vi "solar_voy_def Import (Simple).vi"(4 "Default ID":u16, 5 "Endian (BIG)":enum8{"BIG", "LITTLE"}(ring), 6 "Suppress Errors? (T)":bool=TRUE, 7 "CMD":enum8{"CMD", "TLM"}(ring), 8 "error in (no error)":errorcluster, 9 "ITEMS (Simple)":T6[](array[typedef]), 10 "PACKET":string, 11 "TARGET":string) -> (0 "error out":errorcluster, 3 "PACKET":T1 {"last_time" format="%<%H:%M:%S%3u %m/%d/%y>T"})   [LabVIEW 2018]
uses:
  solar_voy_def_ctl MODIFIERS CONVERSION.ctl
  solar_voy_def_ctl MODIFIERS STATE.ctl
  solar_voy_def_ctl MODIFIERS UNITS.ctl
  solar_voy_def_ctl MODIFIERS LIMITS.ctl
  solar_voy_def_ctl MODIFIERS.ctl
  type/solar_type Item Type.ctl
  solar_voy_def_ctl ITEM TYPE.ctl
  solar_voy_def_ctl ITEM.ctl
  solar_voy_def_ctl PACKET_ID.ctl
  solar_voy_def_ctl PACKET.ctl
  solar_voy_def_ctl ITEM (Simple).ctl
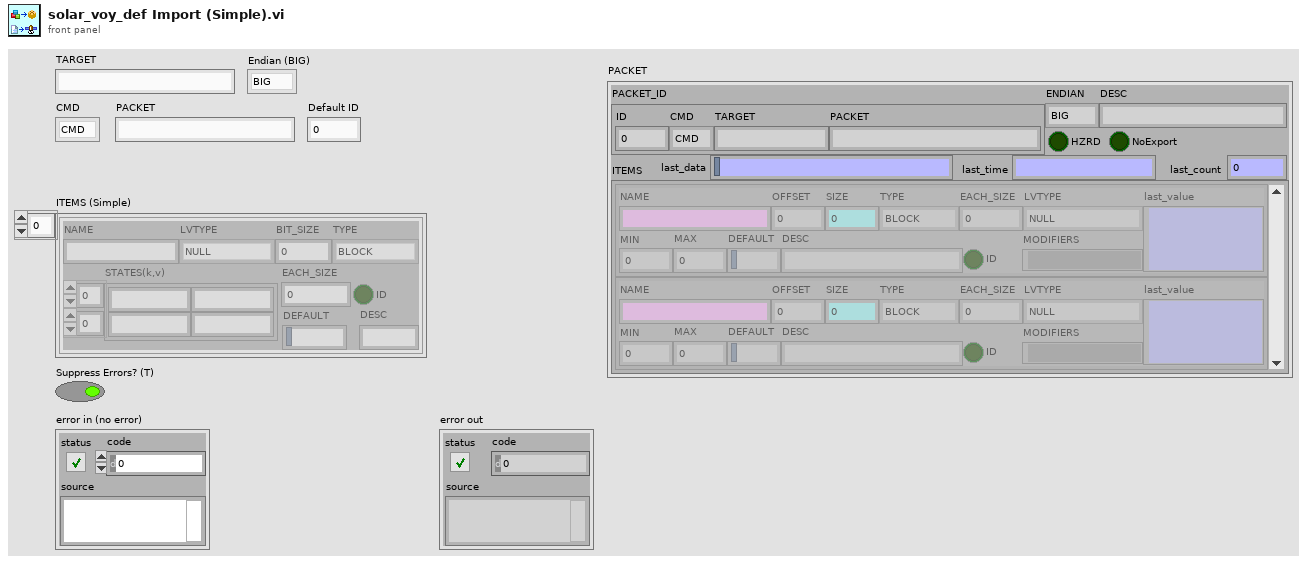
[diagram p1: front panel]
types:
  T1 = typedef "solar_voy_def_ctl PACKET.ctl" = cluster{"PACKET_ID":T2, "ENDIAN":enum8{"BIG", "LITTLE"}, "DESC":string, "HZRD":bool, "ITEMS":T3[], "NoExport":bool, "last_time":timestamp, "last_count":u32, "last_data":string}
  T2 = typedef "solar_voy_def_ctl PACKET_ID.ctl" = cluster{"ID":u16, "CMD":enum8{"CMD", "TLM"}, "TARGET":string, "PACKET":string}
  T3 = typedef "solar_voy_def_ctl ITEM.ctl" = cluster{"NAME":string, "OFFSET":i32, "SIZE":i32, "TYPE":T4, "EACH_SIZE":i32, "LVTYPE":T5, "MIN":dbl, "MAX":dbl, "DEFAULT":string, "DESC":string, "ID":bool, "MODIFIERS":variant, "last_value":variant}
  T4 = typedef "solar_voy_def_ctl ITEM TYPE.ctl" = enum8{"BLOCK", "INT", "UINT", "FLOAT", "STRING"}
  T5 = typedef "solar_type Item Type.ctl" = enum16{"NULL", "UNKNOWN", "CLUSTER", "I8", "I16", "I32", "I64", "U8", "U16", "U32", "U64", "U8_ENUM", "U16_ENUM", "U32_ENUM", "SGL", "DBL", "BOOLEAN", "STRING", "PATH", "VISA", "TAG", "TIME", "I8_1D", "I16_1D", "I32_1D", "I64_1D", "U8_1D", "U16_1D", "U32_1D", "U64_1D", "U8_ENUM_1D", "U16_ENUM_1D", "U32_ENUM_1D", "SGL_1D", "DBL_1D", "BOOLEAN_1D", "STRING_1D", "PATH_1D", "VISA_1D", "TAG_1D", "TIME_1D", "I8_2D", "I16_2D", "I32_2D", "I64_2D", "U8_2D", "U16_2D", "U32_2D", "U64_2D", "U8_ENUM_2D", "U16_ENUM_2D", "U32_ENUM_2D", "SGL_2D", "DBL_2D", "BOOLEAN_2D", "STRING_2D", "PATH_2D", "VISA_2D", "TAG_2D", "TIME_2D"}
  T6 = typedef "solar_voy_def_ctl ITEM (Simple).ctl" = cluster{"NAME":string, "LVTYPE":T5, "BIT_SIZE":i32, "TYPE":T4, "DEFAULT":string, "EACH_SIZE":i32, "ID":bool, "STATES(k,v)":string[][], "DESC":string}
  T7 = typedef "solar_voy_def_ctl MODIFIERS.ctl" = cluster{"LIMITS":T8, "UNITS":T9, "STATES":T10[], "CONVERSION":T11, "FORMAT":string, "REQUIRED":bool, "META":string[][]}
  T8 = typedef "solar_voy_def_ctl MODIFIERS LIMITS.ctl" = cluster{"NAME":string, "PERSIST":i32, "EN":bool, "RED_LO":dbl, "YEL_LO":dbl, "YEL_HI":dbl, "RED_HI":dbl, "GRN_LO":dbl, "GRN_HI":dbl, "FILENAME":string, "ARGS":string}
  T9 = typedef "solar_voy_def_ctl MODIFIERS UNITS.ctl" = cluster{"FULL":string, "ABV":string}
  T10 = typedef "solar_voy_def_ctl MODIFIERS STATE.ctl" = cluster{"KEY":string, "VALUE":string, "COLOR":string, "DESC":string, "HZRD":bool}
  T11 = typedef "solar_voy_def_ctl MODIFIERS CONVERSION.ctl" = cluster{"GENERIC":string, "FILENAME":string, "ARGS":string, "POLYS":cluster{"SEG":bool, "POLY":dbl[]}[]}
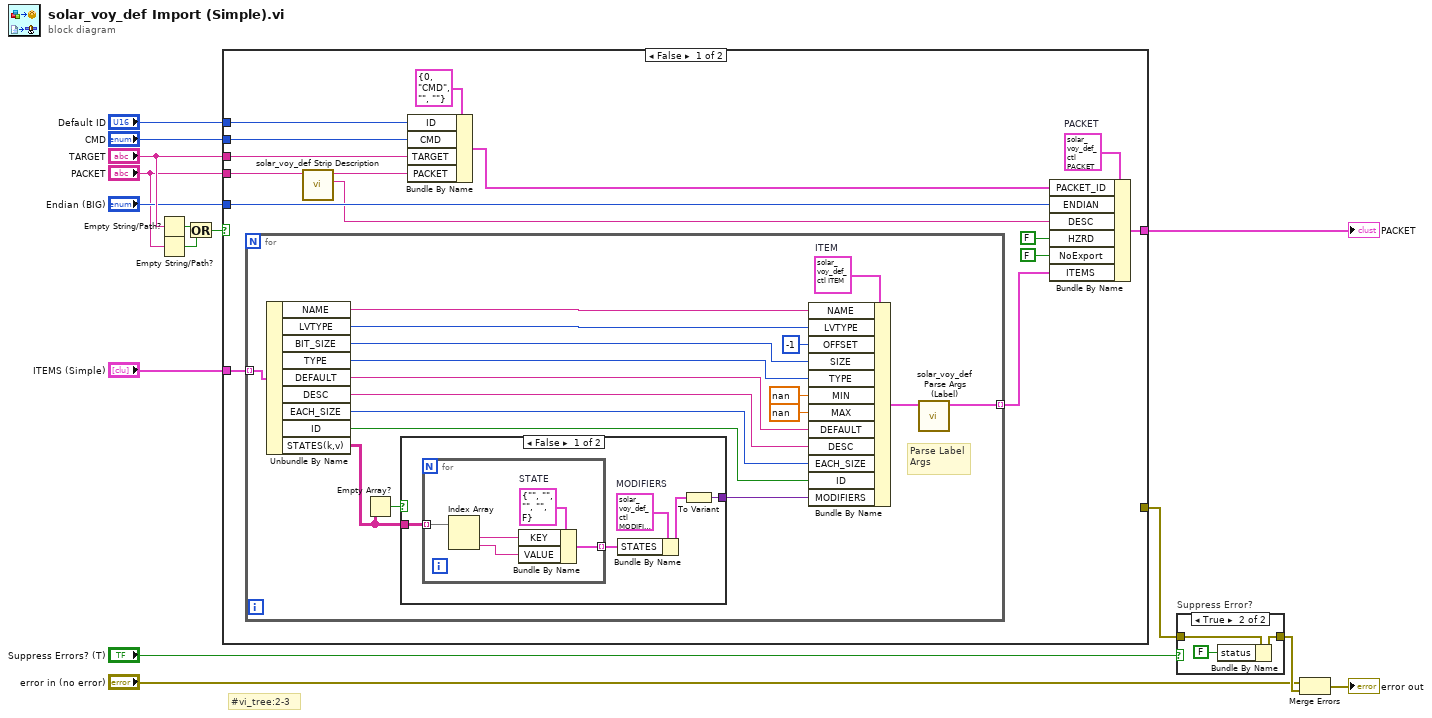
[diagram p0: block diagram]
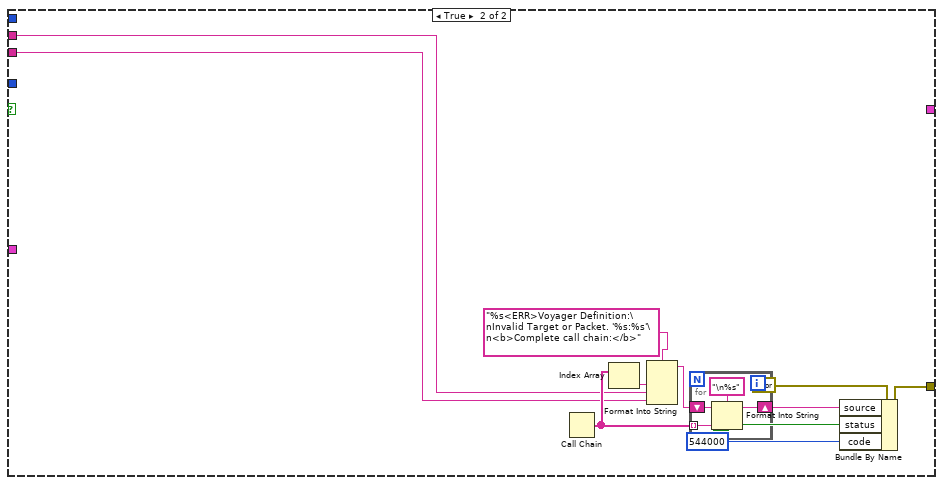
[diagram p3: hidden frame]
diagram:
  # "#vi_tree:2-3"
  n1 = Empty String/Path?(string/path="TARGET") -> (empty?=w12:bool)
  n2 = Empty String/Path?(string/path="PACKET") -> (empty?=w11:bool)
  n3 = Or(x=w12, y=w11) -> (x .or. y?=w10:bool)
  n4 = case shown="False" w10 {
    tunnel: "ITEMS (Simple)" -> [w30 _]
    tunnel: [w29 _] -> w14
    tunnel: "Endian (BIG)" -> [w28 _]
    tunnel: "Default ID" -> [w21 _]
    tunnel: "CMD" -> [w20 _]
    tunnel: "TARGET" -> [w19 w60]
    tunnel: "PACKET" -> [w18 w59]
    tunnel: [_ w61] -> w7
    frame False {
      w25 = T1 {"PACKET_ID"={"ID"=0, "CMD"=enum."CMD", "TARGET"="", "PACKET"=""}, "ENDIAN"=enum."BIG", "DESC"="", "HZRD"=FALSE, "ITEMS"=[], "NoExport"=FALSE, "last_time"=timestamp(0 s since 1904-01-01), "last_count"=0, "last_data"=""}  # PACKET
      n5 = for {
        tunnel: [w34] -> w27 mode=indexing
        tunnel: w30 -> [w48] mode=indexing
        w37 = T3 {"NAME"="", "OFFSET"=0, "SIZE"=0, "TYPE"=enum."BLOCK", "EACH_SIZE"=0, "LVTYPE"=enum."NULL", "MIN"=0.0, "MAX"=0.0, "DEFAULT"="", "DESC"="", "ID"=FALSE, "MODIFIERS"=variant, "last_value"=variant}  # ITEM
        # "Parse Label\nArgs"
        n6 = Unbundle By Name(w48) -> ("NAME"=w36:string, "LVTYPE"=w47:T5, "BIT_SIZE"=w39:i32, "TYPE"=w40:T4, "DEFAULT"=w46:string, "DESC"=w31:string, "EACH_SIZE"=w44:i32, "ID"=w45:bool, "STATES(k,v)"=w33:string[][])
        n7 = Empty Array?(array=w33) -> (empty?=w32:bool)
        n8 = case shown="False" w32 {
          tunnel: w33 -> [w53 _]
          tunnel: [w49 _] -> w38
          frame False {
            w50 = T7 {"LIMITS"={"NAME"="", "PERSIST"=0, "EN"=FALSE, "RED_LO"=0.0, "YEL_LO"=0.0, "YEL_HI"=0.0, "RED_HI"=0.0, "GRN_LO"=0.0, "GRN_HI"=0.0, "FILENAME"="", "ARGS"=""}, "UNITS"={"FULL"="", "ABV"=""}, "STATES"=[], "CONVERSION"={"GENERIC"="", "FILENAME"="", "ARGS"="", "POLYS"=[]}, "FORMAT"="", "REQUIRED"=FALSE, "META"=[]}  # MODIFIERS
            n9 = for {
              tunnel: [w57] -> w52 mode=indexing
              tunnel: w53 -> [w56] mode=indexing
              w58 = T10 {"KEY"="", "VALUE"="", "COLOR"="", "DESC"="", "HZRD"=FALSE}  # STATE
              n10 = Index Array(array=w56) -> (element #1=w55:string, element #2=w54:string)  [unwired: 2 in]
              n11 = Bundle By Name(cluster=w58, "KEY"=w55, "VALUE"=w54) -> (w57:T10)
            }
            n12 = Bundle By Name(cluster=w50, "STATES"=w52) -> (w51:T7)
            n13 = To Variant(anything=w51) -> (Variant=w49:variant)
          }
          frame True {
          }
        }
        n14 = Bundle By Name(cluster=w37, "NAME"=w36, "LVTYPE"=w47, "OFFSET"=-1, "SIZE"=w39, "TYPE"=w40, "MIN"=nan, "MAX"=nan, "DEFAULT"=w46, "DESC"=w31, "EACH_SIZE"=w44, "ID"=w45, "MODIFIERS"=w38) -> (w35:T3)
        n15 = call "solar_voy_def Parse Args (Label).vi"("Default ITEM"=w35) -> ("ITEM out"=w34:T3)  [unwired: 10 in]
      }
      n16 = call "solar_voy_def Strip Description.vi"("Name String"=w18) -> ("Description"=w16:string, "Fixed Name"=w17:string)  [unwired: 9 in]
      n17 = Bundle By Name(cluster=T2 {"ID"=0, "CMD"=enum."CMD", "TARGET"="", "PACKET"=""} ("PACKET_ID"), "ID"=w21, "CMD"=w20, "TARGET"=w19, "PACKET"=w17) -> (w22:T2)
      n18 = Bundle By Name(cluster=w25, "PACKET_ID"=w22, "ENDIAN"=w28, "DESC"=w16, "HZRD"=FALSE, "NoExport"=FALSE ("Do Not Export? (F)"), "ITEMS"=w27) -> (w29:T1)
    }
    frame True {
      n19 = Call Chain() -> (call chain=w64:string[])
      n20 = Index Array(array=w64) -> (element=w66:string)  [unwired: 1 in]
      n21 = Format Into String(format string="%s<ERR>Voyager Definition:\nInvalid Target or Packet. '%s:%s'\n<b>Complete call chain:</b>", w66, w60, w59) -> (resulting string=w65:string)  [unwired: 2 in, 1 out]
      n22 = for {
        tunnel: w64 -> [w73] mode=indexing
        shift-right: [w72] -> w63
        shift-left: w65 -> [w71]
        n23 = Format Into String(format string="\n%s", initial string=w71, w73) -> (resulting string=w72:string)  [unwired: 1 in, 1 out]
      }
      n24 = Bundle By Name(cluster=errorcluster {"status"=FALSE, "code"=0, "source"=""} ("error in (no error)"), "source"=w63, "status"=TRUE, "code"=544000 ("Code")) -> (w61:errorcluster)
    }
  }
  "PACKET" <- w14
  n25 = case "Suppress Error?" shown="True" "Suppress Errors? (T)" {
    tunnel: w7 -> [w74 w77]
    tunnel: [w74 w76] -> w9
    frame False {
    }
    frame True {
      n26 = Bundle By Name(cluster=w77, "status"=FALSE) -> (w76:errorcluster)
    }
  }
  n27 = Merge Errors("error in (no error)", w9) -> (→"error out":errorcluster)
